vi "Convert CAN message to String (RX and TX).vi"(11 "CAN message":T1) -> (3 "CAN":string)   [LabVIEW 2025]
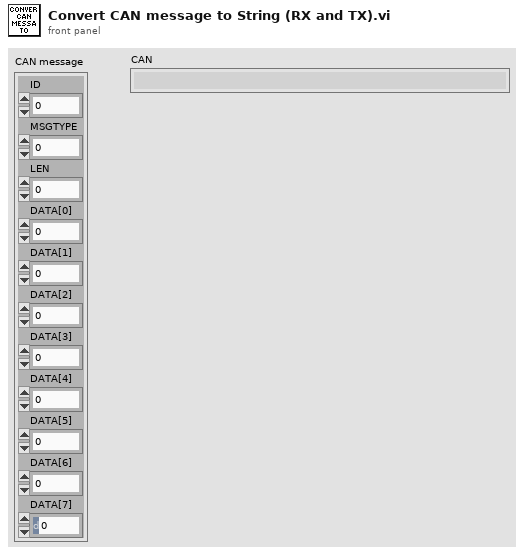
[diagram p1: front panel]
types:
  T1 = cluster{"ID":u32, "MSGTYPE":u8, "LEN":u8, "DATA[0]":u8, "DATA[1]":u8, "DATA[2]":u8, "DATA[3]":u8, "DATA[4]":u8, "DATA[5]":u8, "DATA[6]":u8, "DATA[7]":u8}
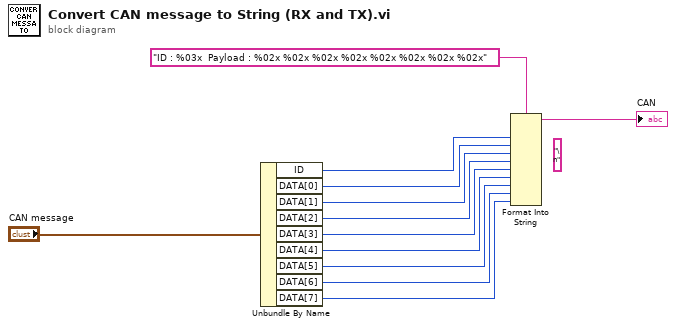
[diagram p0: block diagram]
diagram:
  (unwired) "\n"
  n1 = Unbundle By Name("CAN message") -> ("ID"=w10:u32, "DATA[0]"=w9:u8, "DATA[1]"=w8:u8, "DATA[2]"=w7:u8, "DATA[3]"=w6:u8, "DATA[4]"=w5:u8, "DATA[5]"=w4:u8, "DATA[6]"=w3:u8, "DATA[7]"=w2:u8)
  n2 = Format Into String(format string="ID : %03x  Payload : %02x %02x %02x %02x %02x %02x %02x %02x", w10, w9, w8, w7, w6, w5, w4, w3, w2) -> (resulting string=→"CAN":string)  [unwired: 2 in, 1 out]
